vi "Get Excel All Sheetnames.vi"(8 "error in (no error)":errorcluster, 10 "Path":path, 11 "ExcelReader in":refnum<class "ExcelReader.lvclass">) -> (0 "error out":errorcluster, 2 "SheetNames(\"\")":string[](array[string]), 3 "ExcelReader out":refnum<class "ExcelReader.lvclass">)   [LabVIEW 2015, in "Admin_Actor.lvlib" / "ExcelReader.lvclass"]
uses:
  ExcelReader.lvclass
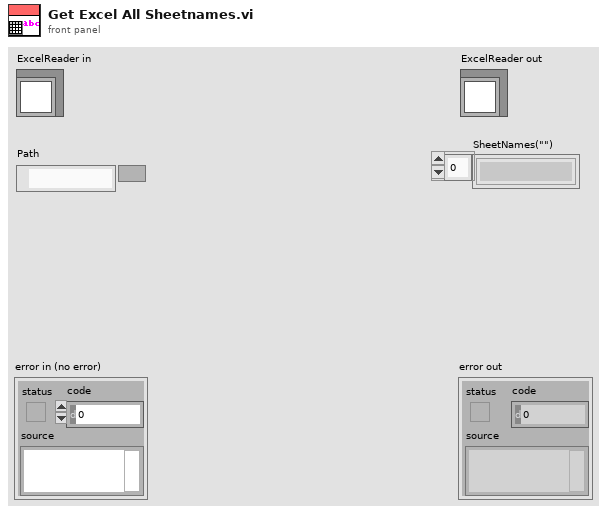
[diagram p1: front panel]
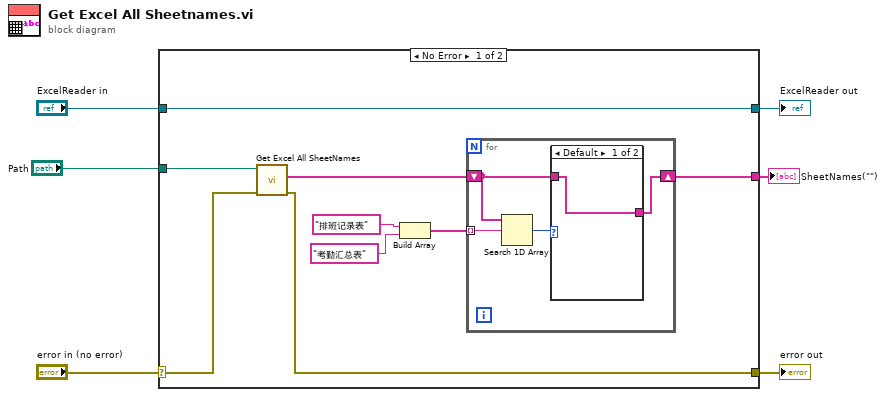
[diagram p0: block diagram]
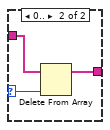
[diagram p2: hidden frame]
diagram:
  n1 = case shown="No Error" "error in (no error)" {
    selector: "error in (no error)" -> [w13 w25]
    tunnel: [w12 w25] -> w5
    tunnel: [w15 w24] -> w3
    tunnel: "ExcelReader in" -> [w15 w24]
    tunnel: "Path" -> [w14 _]
    tunnel: [w7 _] -> w1
    frame No Error {
      n2 = call "Get Excel All SheetNames.vi"("error in (no error)"=w13, "path"=w14) -> ("error out"=w12:errorcluster, "SheetNames(\"\")"=w8:string[])  [unwired: 8 in]
      n3 = Build Array("排班记录表" ("element"), "考勤汇总表" ("element")) -> (w9:string[])
      n4 = for {
        tunnel: w9 -> [w19] mode=indexing
        shift-right: [w16] -> w7
        shift-left: w8 -> [w17]
        n5 = Search 1D Array(1D array=w17, element=w19) -> (index of element=w18:i32)  [unwired: 1 in]
        n6 = case shown="Default" w18 {
          selector: w18 -> [_ w22]
          tunnel: w17 -> [w20 w23]
          tunnel: [w20 w21] -> w16
          frame Default {
          }
          frame 0.. {
            n7 = Delete From Array(array=w23, index=w22) -> (array with subset deleted=w21:string[])  [unwired: 1 in, 1 out]
          }
        }
      }
    }
    frame Error {
    }
  }
  "error out" <- w5
  "ExcelReader out" <- w3
  "SheetNames(\"\")" <- w1
